vi "GetCurrent.vi"(4 "error in":errorcluster, 5 "connection ID":refnum<k5>) -> (0 "Current":string, 1 "error out":errorcluster, 2 "connection ID out":refnum<k5>, 3 "Answer":bool)   [LabVIEW 2013]
uses:
  <vilib>/regexp/Match Regular Expression.xnode
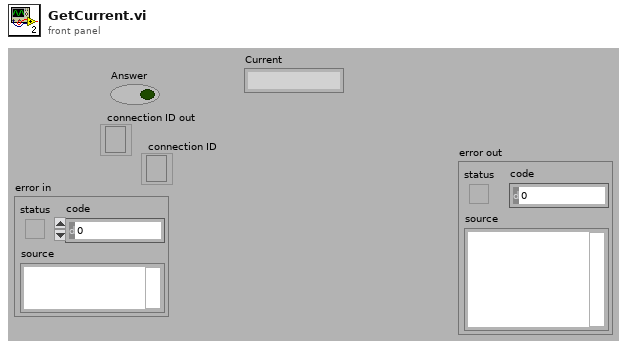
[diagram p1: front panel]
types:
  T1 = enum16{"Standard", "Buffered", "CRLF", "Immediate"}
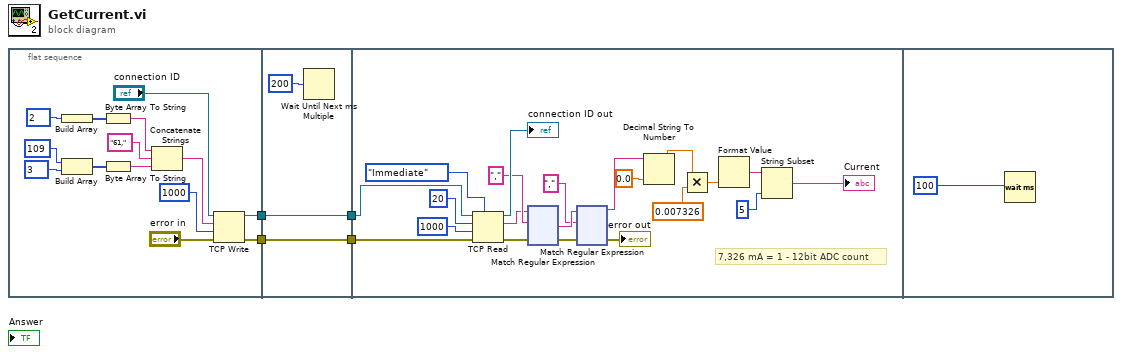
[diagram p0: block diagram]
diagram:
  n1 = flat-sequence {
    tunnel: [w15] -> w3
    tunnel: [w14] -> w1
    tunnel: [w20] -> w4
    tunnel: w3 -> [w20]
    tunnel: [w19] -> w2
    tunnel: w1 -> [w19]
    tunnel: w4 -> [w38]
    tunnel: w2 -> [w37]
    frame #0 {
      n2 = Build Array(u8 2 ("y")) -> (w11:u8[])
      n3 = Build Array(u8 109 ("y"), u8 3 ("y")) -> (w7:u8[])
      n4 = Byte Array To String(unsigned byte array=w11) -> (string=w10:string)
      n5 = Byte Array To String(unsigned byte array=w7) -> (string=w6:string)
      n6 = Concatenate Strings(w10, "61," ("string"), w6) -> (w5:string)
      n7 = TCP Write(connection ID="connection ID", data in=w5, error in (no error)="error in", 9:1000 ("timeout ms (25000)")) -> (connection ID out=w15:refnum<k5>, error out=w14:errorcluster)  [unwired: 1 out]
    }
    frame #1 {
      n8 = Wait Until Next ms Multiple(millisecond multiple=u32 200) -> ()  [unwired: 1 out]
    }
    frame #2 {
      # "7,326 mA = 1 - 12bit ADC count"
      n9 = TCP Read(connection ID=w38, bytes to read=20, error in (no error)=w37, 7:T1."Immediate" ("mode (standard)"), 9:1000 ("timeout ms (25000)")) -> (connection ID out=→"connection ID out":refnum<k5>, data out=w30:string, error out=w32:errorcluster)
      n10 = xnode "Match Regular Expression"("input string"=w30, "regular expression"=",", "error in"=w32) -> ("after match"=w35:string, "error out"=w33:errorcluster)  [unwired: 3 in, 3 out]
      n11 = xnode "Match Regular Expression"("input string"=w35, "regular expression"=",", "error in"=w33) -> ("before match"=w25:string, "error out"=→"error out":errorcluster)  [unwired: 3 in, 3 out]
      n12 = Decimal String To Number(string=w25, default (0L)=0.0 ("default (0 I32)")) -> (number=w26:dbl)  [unwired: 1 in, 1 out]
      n13 = Multiply(x=w26, y=0.007326 ("default (0 I32)")) -> (x*y=w27:dbl)
      n14 = Format Value(value (0)=w27) -> (output string=w23:string)  [unwired: 2 in]
      n15 = String Subset(string=w23, length (rest)=5 ("length (rest)")) -> (substring=→"Current":string)  [unwired: 1 in]
    }
    frame #3 {
      n16 = Wait (ms)(milliseconds to wait=u32 100) -> ()  [unwired: 1 out]
    }
  }
